vi "Shutdown Daemon.vi"(8 "error in":errorcluster, 11 "Serial Slave in":refnum<class "Serial Slave.lvclass">) -> (0 "error out":errorcluster)   [LabVIEW 2012, in "Serial Slave.lvclass"]
doc: "This provides an interface for the slave to shut down its protocol daemon."
uses:
  Serial Slave.lvclass
  Network Slave.lvclass
  Serial Slave.lvclass/Serial Slave.ctl
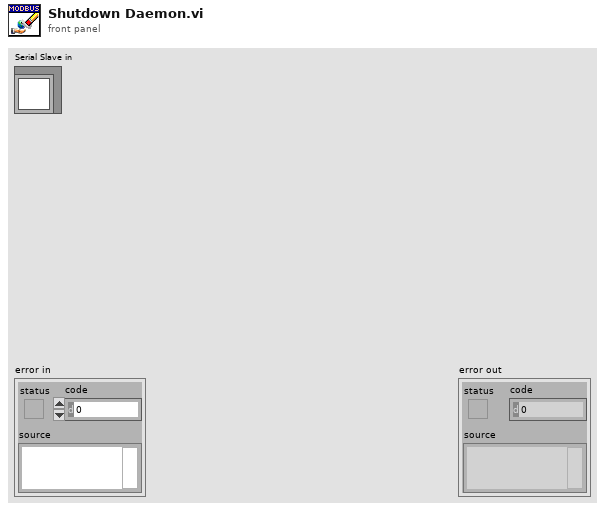
[diagram p1: front panel]
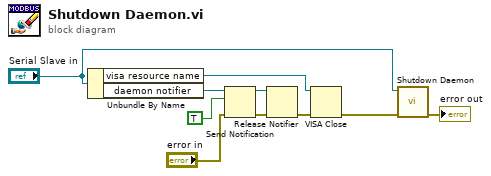
[diagram p0: block diagram]
diagram:
  n1 = Unbundle By Name("Serial Slave in") -> ("visa resource name"=w6:refnum<visa-resource-name>, "daemon notifier"=w7:refnum<notifier>)
  n2 = Send Notification(notification=TRUE, notifier=w7, error in (no error)="error in") -> (notifier out=w9:refnum<notifier>, error out=w8:errorcluster)
  n3 = Release Notifier(notifier=w9, error in (no error)=w8) -> (error out=w5:errorcluster)  [unwired: 1 in, 2 out]
  n4 = VISA Close(VISA resource name=w6, error in (no error)=w5) -> (error out=w1:errorcluster)
  n5 = call-parent "Shutdown Daemon.vi"("error in"=w1, "network slave in"="Serial Slave in") -> ("error out"=→"error out":errorcluster)  [unwired: 9 in]
